vi "Init Base Graph.vi"(6 "Z Scale.Marker Values[]":cluster{"Numeric":dbl, "Numeric":u32}[](array[cluster]), 8 "error in (no error)":errorcluster, 9 "Sizes":cluster{"Height":u32, "Width":u32}, 10 "IntGraph Ref":refnum<vi>, 11 "TG Base Graph in":refnum<class "TG Base Graph.lvclass">) -> (0 "error out":errorcluster, 3 "TG Base Graph out":refnum<class "TG Base Graph.lvclass">)   [LabVIEW 2023, in "TG Base Graph.lvclass"]
uses:
  TG Base Graph.lvclass
  TG Base Graph.lvclass/TG Base Graph.ctl
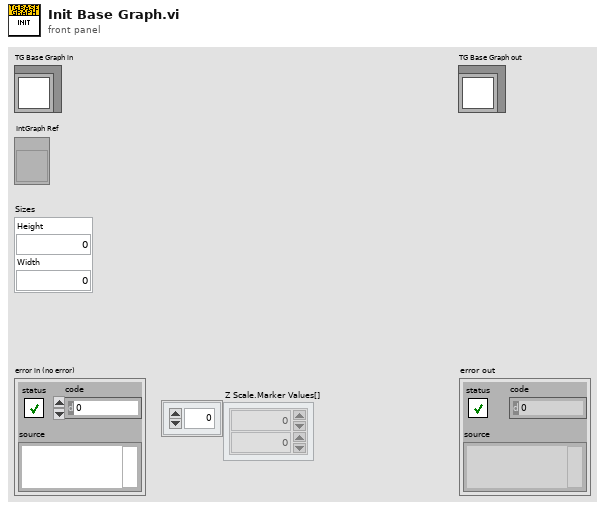
[diagram p1: front panel]
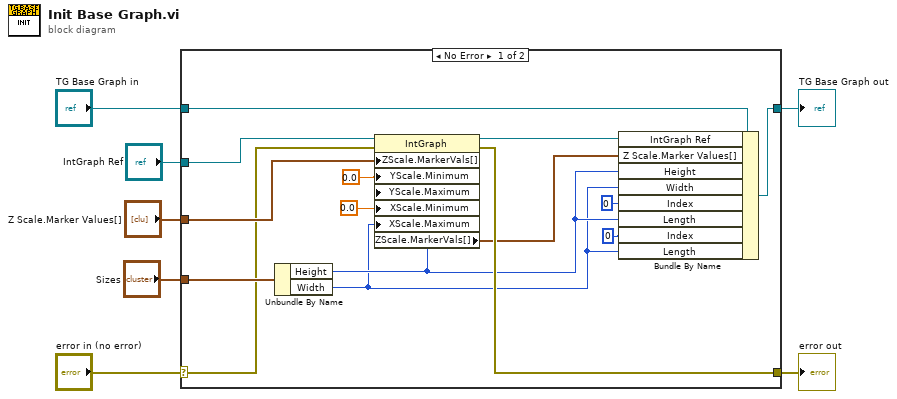
[diagram p0: block diagram]
diagram:
  n1 = case shown="No Error" "error in (no error)" {
    selector: "error in (no error)" -> [w16 w24]
    tunnel: [w15 w24] -> w6
    tunnel: [w21 w23] -> w4
    tunnel: "TG Base Graph in" -> [w22 w23]
    tunnel: "IntGraph Ref" -> [w20 _]
    tunnel: "Z Scale.Marker Values[]" -> [w18 _]
    tunnel: "Sizes" -> [w17 _]
    frame No Error {
      n2 = Unbundle By Name(w17) -> ("Height"=w9:u32, "Width"=w8:u32)
      n3 = property class="IntGraph"(reference=w20, error in=w16, "ZScale.MarkerVals[]"=w18, "YScale.Minimum"=0.0 ("Y Scale.Range:Minimum"), "YScale.Maximum"=w9, "XScale.Minimum"=0.0 ("X Scale.Range:Minimum"), "XScale.Maximum"=w8) -> (reference out=w19:refnum<vi>, error out=w15:errorcluster, "ZScale.MarkerVals[]"=w12:cluster{dbl, u32}[])
      n4 = Bundle By Name(cluster=w22, "IntGraph Ref"=w19, "Z Scale.Marker Values[]"=w12, "Height"=w9, "Width"=w8, "Index"=u32 0 ("ROI XY.ROI Y.Index"), "Length"=w9, "Index"=u32 0 ("ROI XY.ROI X.Index"), "Length"=w8) -> (w21:refnum<class "TG Base Graph.lvclass">)
    }
    frame Error {
    }
  }
  "error out" <- w6
  "TG Base Graph out" <- w4
